vi "Actor Core.vi"(8 "error in":errorcluster, 11 "Nested in":refnum<class "Model_AMC.lvclass">) -> (0 "error out":errorcluster, 3 "Actor out":refnum<class "Actor.lvclass">)   [LabVIEW 2021, in "Model_AMC.lvclass"]
doc: "(<B>Filename</B>: Actor Framework.lvlib:Actor.lvclass:Actor Core.vi)\n\nReceives messages to the actor, reacts to them, and initiates any error handling that may shut the actor down.\n\nDescendant classes may override this VI to append parallel tasks for the actor to complete while it handles messages. Overrides use the Call Parent Method node."
uses:
  Model_AMC.lvclass
  Model_AMC.lvclass/Model_AMC.ctl
  <vilib>/ActorFramework/Actor/Actor.lvclass
  <vilib>/ActorFramework/Stop Msg/Stop Msg.lvclass
  <userlib>/John_Lib/AMC_FW/AMC_FW.lvlib
  <userlib>/John_Lib/Control/Panel State.ctl
  <userlib>/John_Lib/OPCUA/OPCUA.lvclass
  57b1ff99-141e-4da6-9bdf-70ec06928c0d.vi
  14795f1b-d0b1-44de-8d07-189a26e8dea2.vi
  C:/Program Files (x86)/National Instruments/LabVIEW 2021/user.lib/John_Lib/AbstractActorTemplate/AbstractActorTemplate/UIActorTop.lvclass
  C:/Program Files (x86)/National Instruments/LabVIEW 2021/vi.lib/ActorFramework/Actor/Actor.lvclass
  C:/Program Files (x86)/National Instruments/LabVIEW 2021/project/Create Actor from Template/_Model_AMC/Model_AMC.lvclass
  6f5781f2-676e-4ccc-9b4e-d2ad4bb5011c.vi
  <userlib>/John_Lib/AbstractActorTemplate/AbstractActorTemplate/UIActorTop.lvclass
  dd6ce886-d6bc-4aa3-89ad-92228f1f1005.vi
  eab6dcde-6998-4829-8205-257228226865.vi
  bac1cae5-b367-464c-b2b6-145fd5ecb0f6.vi
  TopRef.ctl
  b524a0ae-aab8-42c6-9847-114de1d87e8e.vi
panel:
  in  "Close":bool
  in  "Initialize":bool
  out "Close OK status":bool
  out "Initialize OK status":bool
  out "Messages":string
  out "Read Error":bool
  out "ReadIndex":u32
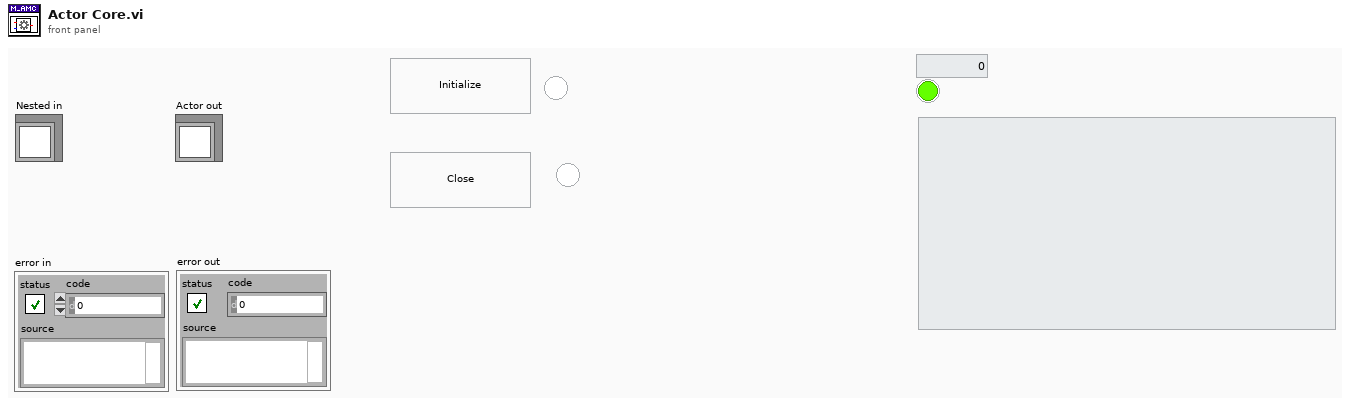
[diagram p1: front panel]
types:
  T1 = typedef "Model_AMC.lvclass/TopRef.ctl" = cluster{"Self ActorVI Ref":refnum<vi>}
  T2 = typedef "OPCUA.lvlib/OPCUA.lvclass/OPCUA Even.ctl" = cluster{"OPC UA data change":refnum<user-event>, "ReSubscribtion":refnum<user-event>}
  T3 = cluster{"Stop":refnum<user-event>, "Messages":refnum<user-event>}
  T4 = typedef "AMC_FW.lvlib/Queue.ctl" = cluster{"Q":T5, "Name":string}
  T5 = typedef "AMC_FW.lvlib/Message Queue.ctl" = refnum<queue>
  T6 = typedef "Panel State.ctl" = string
  T7 = typedef "Model_AMC.lvclass/DVR.ctl" = cluster{"JKI_Network_Streams":refnum<class "NetworkConnection.lvclass">, "AMC Q":T8, "Connnected":bool}
  T8 = typedef "Model_AMC.lvclass/AMC Q.ctl" = cluster{"Main":T4, "OPCUA":T4, "NetworkSteam":T4}
  T9 = typedef "AMC_FW.lvlib/Reply Data Type.ctl" = cluster{"Message Type":T10, "Data":variant}
  T10 = typedef "AMC_FW.lvlib/Message Type.ctl" = enum16{"Normal", "AMC_Reply", "OPCUA", "NetworkSteam"}
  T11 = typedef "Subscription Data Change.ctl" = cluster{"node ID":T12, " value":variant, "timestamp":timestamp, "data type":T13, "status code":T14}
  T12 = typedef "NodeId.ctl" = string
  T13 = typedef "Data Type.ctl" = u16
  T14 = typedef "OPC UA StatusCode.ctl" = u32
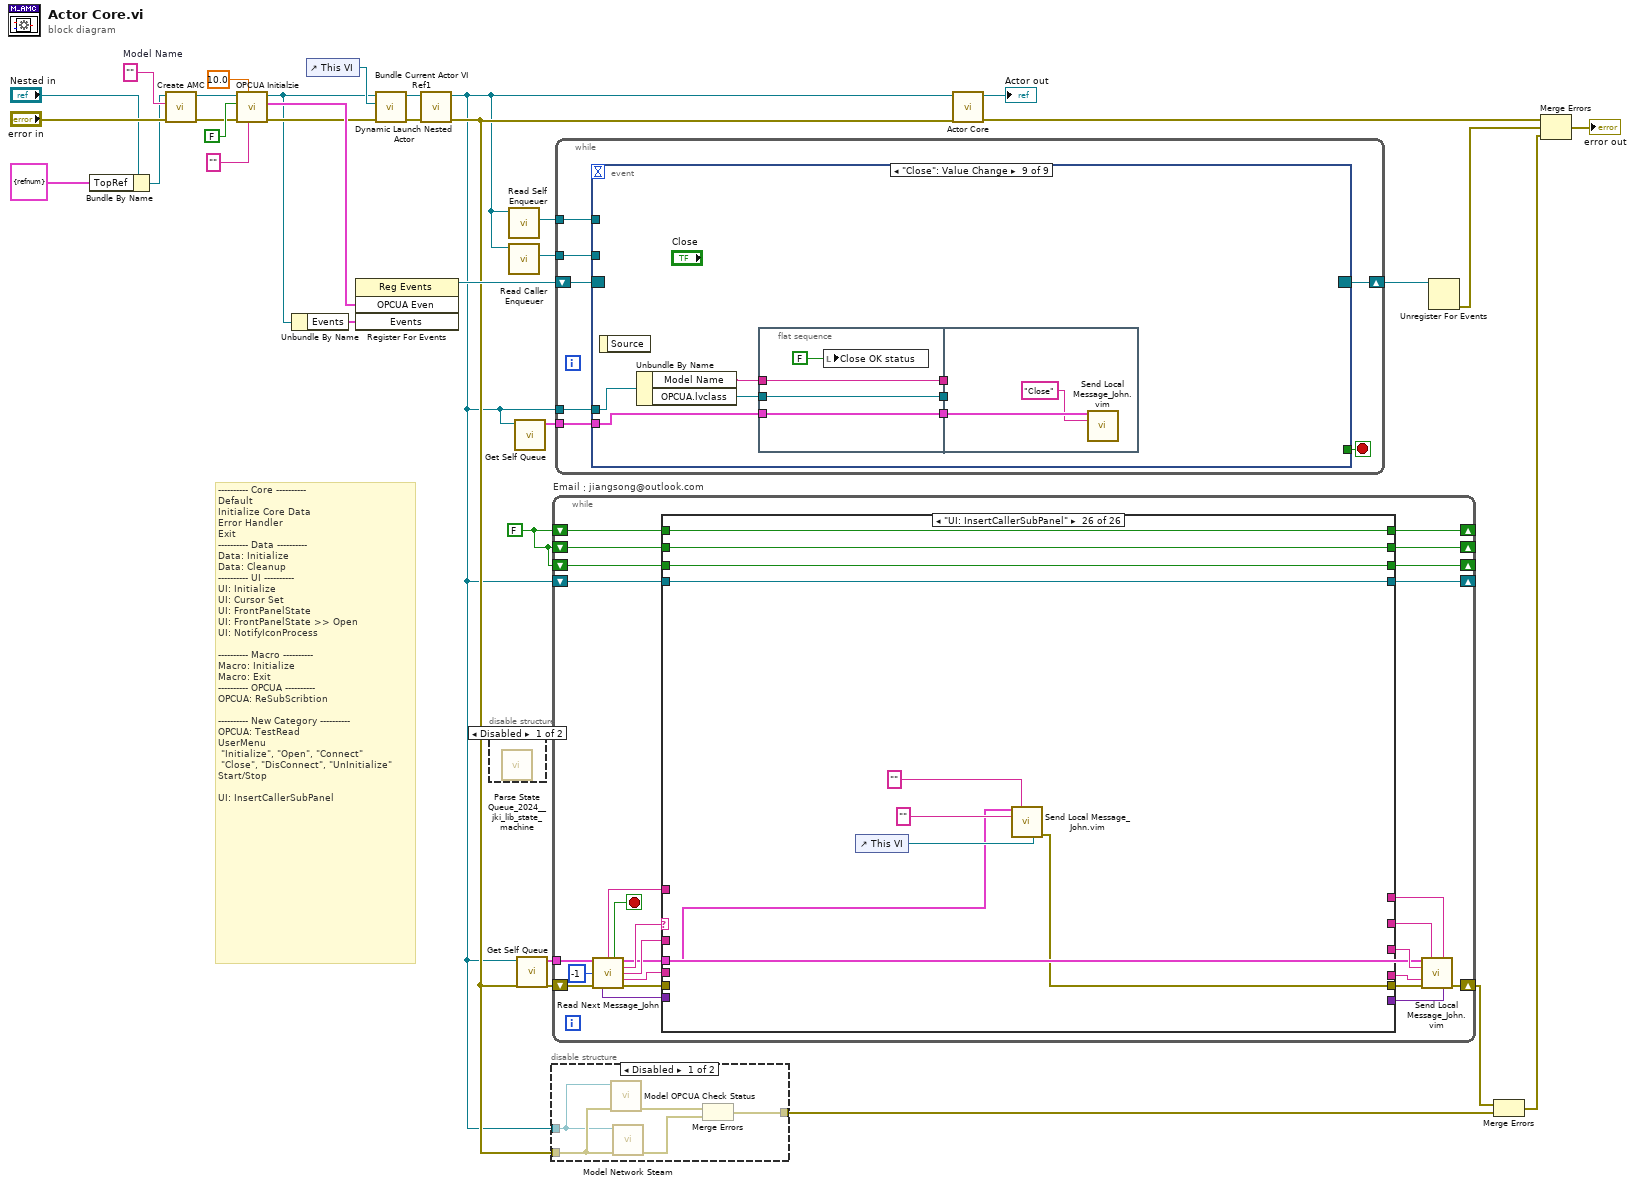
[diagram p0: block diagram]
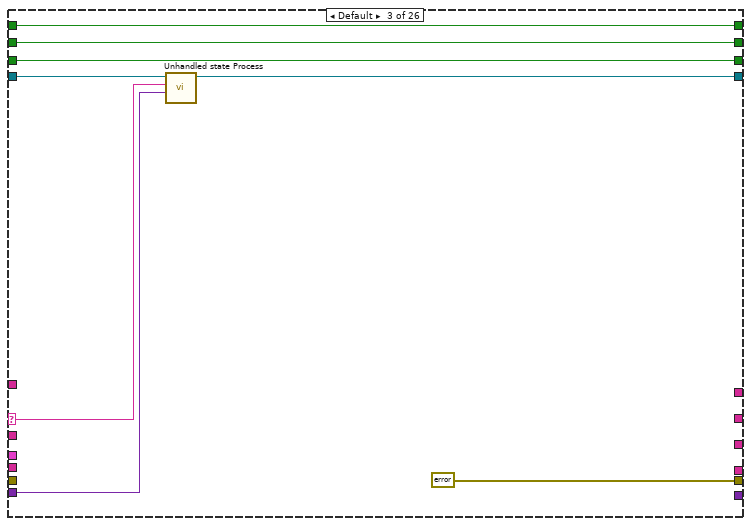
[diagram p6: hidden frame]
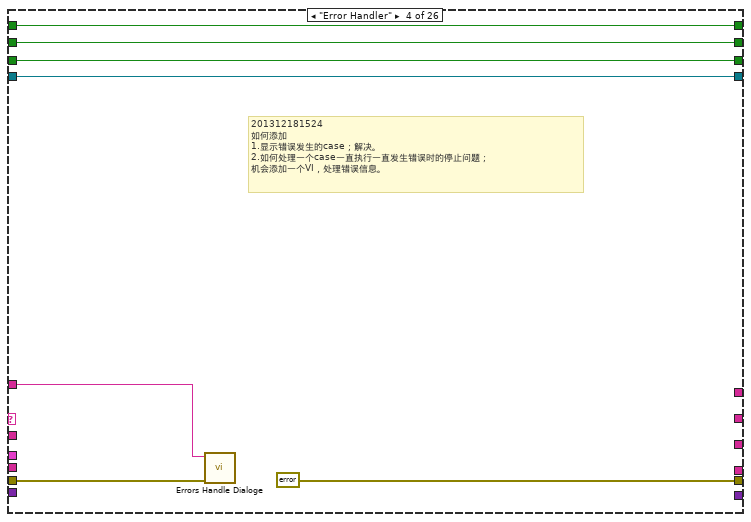
[diagram p7: hidden frame]
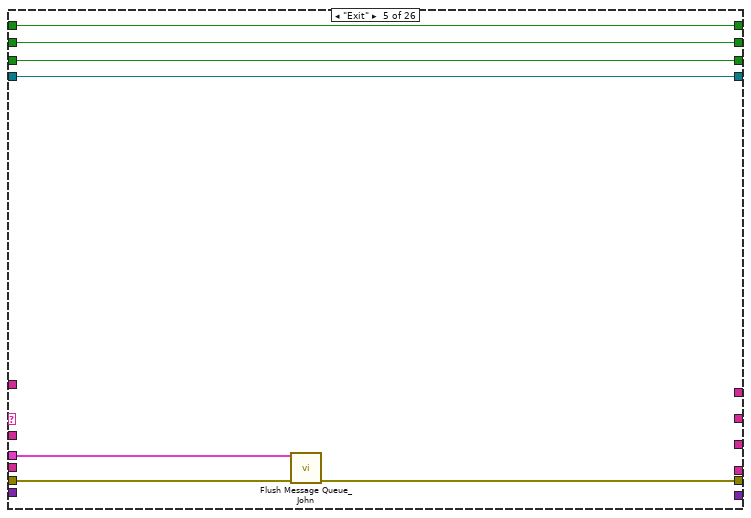
[diagram p8: hidden frame]
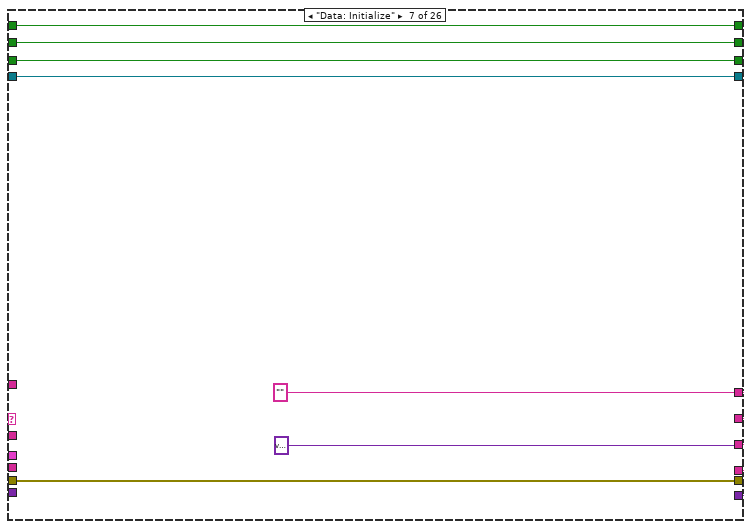
[diagram p10: hidden frame]
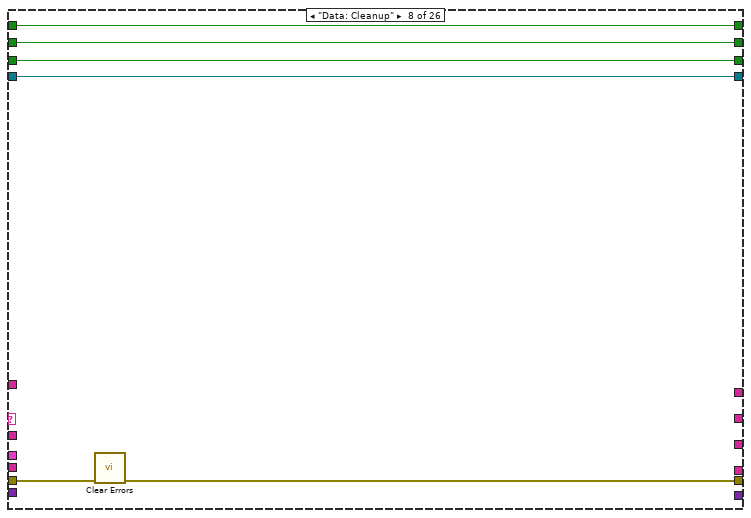
[diagram p11: hidden frame]
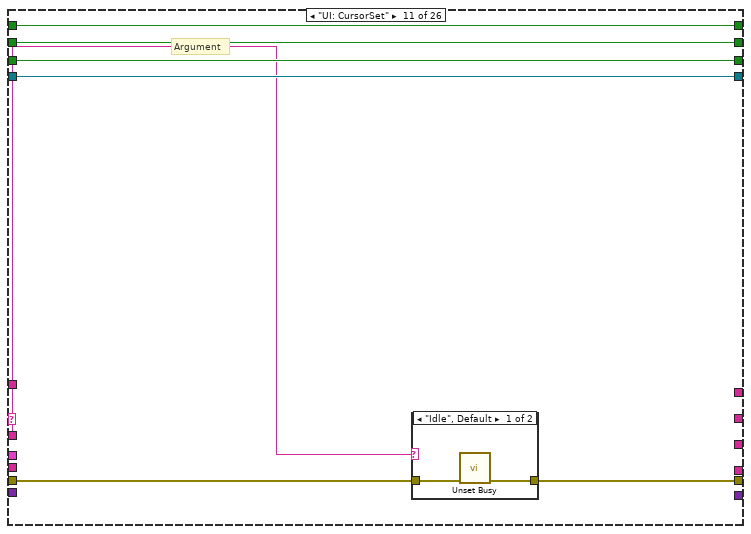
[diagram p14: hidden frame]
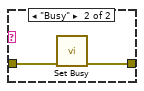
[diagram p15: hidden frame]
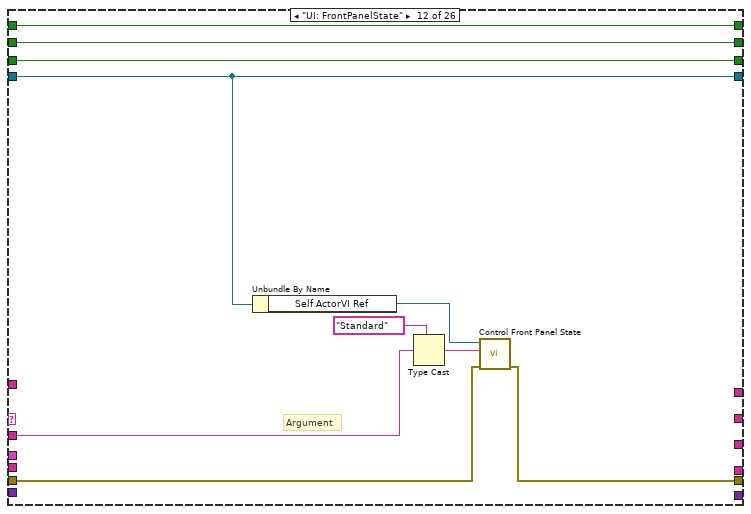
[diagram p16: hidden frame]
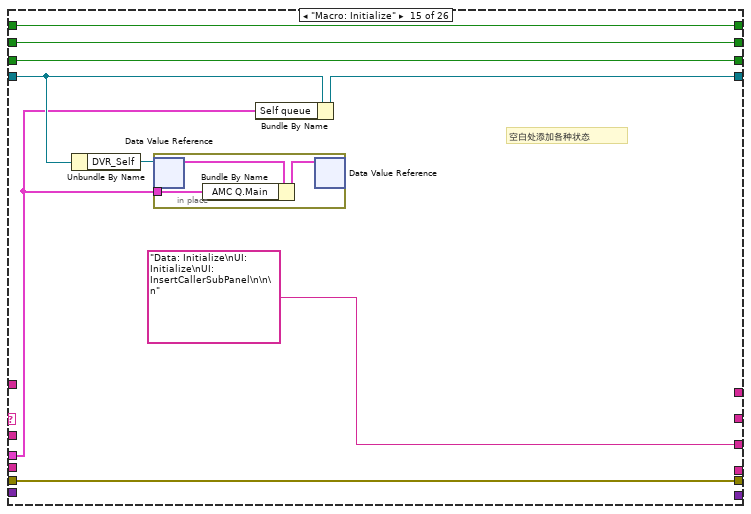
[diagram p19: hidden frame]
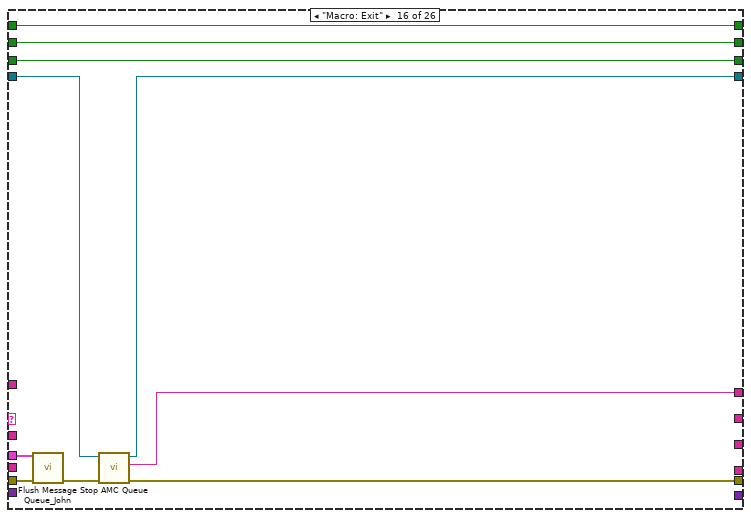
[diagram p20: hidden frame]
diagram:
  w18 = ""  # Model Name
  w25 = FALSE
  # "---------- Core ----------\nDefault\nInitialize Core Data\nError Handler\nExit\n---------- Data ----------\nData: Initialize\nData: Cleanup\n---------- UI ----------\nUI: Initialize\nUI: Cursor Set\nUI: FrontPanelState\nUI: FrontPanelState >> Open\nUI: NotifyIconProcess\n\n---------- Macro ----------\nMacro: Initialize\nMacro: Exit\n---------- OPCUA ----------\nOPCUA: ReSubScribtion\n\n---------- New Category ----------\nOPCUA: TestRead\nUserMenu\n \"Initialize\", \"Open\", \"Connect\" \n \"Close\", \"DisConnect\", \"UnInitialize\" \nStart/Stop\n\nUI: InsertCallerSubPanel"
  n1 = Bundle By Name(cluster="Nested in", "TopRef"=T1 {"Self ActorVI Ref"=refnum}) -> (w1:refnum<class "Model_AMC.lvclass">)
  n2 = call "Create AMC.vi"("error in (no error)"="error in", "message queue name"=w18, "Model_AMC in"=w1) -> ("error out"=w19:errorcluster, "Model_AMC out"=w21:refnum<class "Model_AMC.lvclass">)  [unwired: 7 in]
  n3 = call "OPCUA Initialzie.vi"("SUbscription Node IDs"="", "publishing interval (10 ms)"=10.0, "error in (no error)"=w19, "OPCUA Initialize"=FALSE, "Model_AMC in"=w21) -> ("error out"=w6:errorcluster, "OPCUA Even"=w17:T2, "Model_AMC out"=w3:refnum<class "Model_AMC.lvclass">)  [unwired: 4 in]
  n4 = Unbundle By Name(w3) -> ("Events"=w9:T3)
  n5 = control-ref of="This VI"() -> (w7:refnum<vi>)
  n6 = register-events ("Main Register for Events")(w17, w9) -> (reference out=w32:refnum<event-registration>)  [unwired: 2 in, 1 out]
  n7 = call "Bundle Current Actor VI Ref1.vi"("error in (no error)"=w6, "This VI"=w7, "Model_AMC in"=w3) -> ("error out"=w5:errorcluster, "Model_AMC out"=w8:refnum<class "Model_AMC.lvclass">)  [unwired: 5 in, 2 out]
  n8 = call-dynamic "Dynamic Launch Nested Actor.vi"("error in (no error)"=w5, "UI ActorTop in"=w8) -> ("error out"=w24:errorcluster, "UI ActorTop out"=w13:refnum<class "Model_AMC.lvclass">)  [unwired: 8 in]
  n9 = disable-structure shown="Disabled" {
    frame Disabled {
      n10 = call <vilib>:"Parse State Queue_2024__jki_lib_state_machine.vi"() -> ()  [unwired: 12 in, 4 out]
    }
    frame Enabled {
    }
  }
  n11 = call <vilib>:"Read Self Enqueuer.vi"("Actor"=w13) -> ("Self Enqueuer"=w27:refnum<class "Message Enqueuer.lvclass">)  [unwired: 10 in]
  n12 = call <vilib>:"Read Caller Enqueuer.vi"("Actor"=w13) -> ("Caller Enqueuer"=w26:refnum<class "Message Enqueuer.lvclass">)  [unwired: 10 in]
  n13 = call "Get Self Queue.vi"("Model_AMC in"=w13) -> ("Self queue"=w12:T4)  [unwired: 10 in]
  n14 = call "Get Self Queue.vi"("Model_AMC in"=w13) -> ("Self queue"=w22:T4)  [unwired: 10 in]
  n15 = disable-structure shown="Disabled" {
    disable-tunnel: w24 -> [w38 _]
    disable-tunnel: w13 -> [w37 _]
    disable-tunnel: [w34 _] -> w16
    frame Disabled {
      n16 = call "Model OPCUA Check Status.vi"("error in (no error)"=w38, "Model_AMC in"=w37) -> ("error out"=w36:errorcluster)  [unwired: 8 in, 1 out]
      n17 = call "Model Network Steam.vi"("error in (no error)"=w38, "Model_AMC in"=w37) -> ("error out"=w35:errorcluster)  [unwired: 8 in, 1 out]
      n18 = Merge Errors(w36, w35) -> (w34:errorcluster)
    }
    frame Enabled {
    }
  }
  n19 = while "Email：jiangsong@outlook.com" {
    shift-right: [w49] -> w15
    shift-left: w24 -> [w58]
    shift-right: [w63] -> _
    shift-left: w25 -> [w64]
    shift-right: [w59] -> _
    shift-left: w13 -> [w52]
    shift-right: [w60] -> _
    shift-left: w25 -> [w50]
    shift-right: [w61] -> _
    shift-left: w25 -> [w62]
    tunnel: w22 -> [w55]
    stop <- w41 stop-if-true
    n20 = call <userlib>:"Read Next Message_John.vi"("Queue In"=w55, "timeout (-1 ms)"=-1, "error in"=w58) -> ("Previous State + Arguments"=w51:string, "exit process?"=w41:bool, "Queue Out"=w40:T4, "Current State"=w56:string, "Arguments"=w54:string, "message value"=w53:string, "variant"=w42:variant, "error out"=w57:errorcluster)  [unwired: 3 in, 2 out]
    n21 = case shown="\"UI: InsertCallerSubPanel\"" w56 {
      selector: w56 -> [_ _ w76 _ _ _ _ _ _ _ _ _ _ _ _ _ _ _ _ _ w206 w223 w242 w256 _ _]
      tunnel: w40 -> [_ _ _ _ w91 _ _ _ _ _ _ _ _ _ w156 w174 _ _ _ _ _ _ _ _ _ w280]
      tunnel: w53 -> [_ _ _ _ _ _ _ _ _ _ _ _ _ _ _ _ _ _ w192 _ w205 w219 _ w255 w269 _]
      tunnel: [w65 w74 errorcluster {"status"=FALSE, "code"=0, "source"=""} ("error out") errorcluster {"status"=FALSE, "code"=0, "source"=""} ("error out") w92 w98 w106 w111 w116 w122 w127 w139 w146 w152 w161 w170 w180 w190 w196 w204 w211 w221 w247 w261 w270 w279] -> w48
      tunnel: w57 -> [w65 w74 _ w84 w93 w98 w106 w109 w116 w122 w128 w140 w146 w152 w161 w173 w180 w190 w196 w204 w207 w226 w243 w257 _ _]
      tunnel: w64 -> [w69 w73 w82 w89 w96 w101 w108 w112 w119 w124 w131 w145 w150 w155 w164 w177 w182 w189 w195 w203 w218 w241 w254 w268 w278 w287]
      tunnel: [w69 w73 w82 w89 w96 w101 w108 w112 w119 w124 w131 w145 w150 w155 w164 w177 w182 w189 w195 w203 w218 w241 w254 w268 w278 w287] -> w63
      tunnel: w62 -> [w68 w72 w81 w86 w95 w100 w107 w114 w118 w120 w130 w144 w149 w154 w163 w175 w181 w188 w194 w202 w217 w240 w253 w267 w277 w286]
      tunnel: w50 -> [w67 w70 w79 w87 w94 w97 w105 w110 w115 w121 w126 w143 w148 w151 w162 w176 w178 w187 w193 w201 w216 w239 w252 w266 w276 w285]
      tunnel: w52 -> [w66 w71 w77 w88 w90 w99 w103 w113 w117 w123 w129 w142 w147 w153 w157 w172 w179 w185 w191 w200 w212 w228 w248 w262 w273 w284]
      tunnel: [w68 w72 w81 w86 w95 w100 w107 w114 w118 w120 w130 w144 w149 w154 w163 w175 w181 w188 w194 w202 w217 w240 w253 w267 w277 w286] -> w61
      tunnel: [w67 w70 w79 w87 w94 w97 w105 w110 w115 w121 w126 w143 w148 w151 w162 w176 w178 w187 w193 w201 w216 w239 w252 w266 w276 w285] -> w60
      tunnel: [w66 w71 w78 w88 w90 w99 w103 w113 w117 w123 w129 w142 w147 w153 w159 w168 w179 w186 w191 w200 w213 w236 w249 w263 w271 w284] -> w59
      tunnel: w54 -> [_ _ _ _ _ _ _ _ _ _ w125 w136 _ _ _ _ _ _ _ _ _ _ _ _ _ _]
      tunnel: w51 -> [_ _ _ w83 _ _ _ _ _ _ _ _ _ _ _ _ _ _ _ _ _ _ _ _ _ _]
      tunnel: [_ _ _ _ _ _ w104 _ _ _ _ _ _ _ _ _ _ _ _ _ _ _ _ _ _ _] -> w47
      tunnel: [_ _ _ _ _ _ w104 _ _ _ _ _ _ _ _ w169 _ _ _ _ _ _ _ _ _ _] -> w46
      tunnel: [_ _ _ _ _ _ w104 _ _ _ _ _ _ _ "Data: Initialize\nUI: Initialize\nUI: InsertCallerSubPanel\n\n\n" _ _ _ _ _ _ w222 _ _ _ _] -> w45
      tunnel: [_ _ _ _ _ _ w104 _ _ _ _ _ _ _ _ _ _ _ _ _ _ _ _ _ _ _] -> w44
      tunnel: [_ _ _ _ _ _ variant ("variant") _ _ _ _ _ _ _ _ _ _ _ _ _ _ _ _ _ _ _] -> w43
      tunnel: w42 -> [_ _ w75 _ _ _ _ _ _ _ _ _ _ _ _ _ _ _ _ _ w215 w238 w251 w265 _ _]
      frame "", "Idle" {
      }
      frame "---------- Core ----------" {
      }
      frame Default {
        n22 = call "Unhandled state Process.vi"("variant"=w75, "Unhandled state Case Name"=w76, "Model_AMC in"=w77) -> ("Model_AMC out"=w78:refnum<class "Model_AMC.lvclass">)  [unwired: 7 in, 1 out]
      }
      frame "Error Handler" {
        # "201312181524\n如何添加\n1.显示错误发生的case；解决。\n2.如何处理一个case一直执行一直发生错误时的停止问题；\n机会添加一个VI，处理错误信息。"
        n23 = call <userlib>:"Errors Handle Dialoge.vi"("error in (no error)"=w84, "Message"=w83) -> ()  [unwired: 8 in, 2 out]
      }
      frame "Exit" {
        n24 = call <userlib>:"Flush Message Queue_John.vi"("Queue In"=w91, "error in"=w93) -> ("error out"=w92:errorcluster)  [unwired: 11 in, 2 out]
      }
      frame "---------- Data ----------" {
      }
      frame "Data: Initialize" {
        w104 = "" ("Elements in Front")
      }
      frame "Data: Cleanup" {
        n25 = call <vilib>:"Clear Errors.vi"("error in (no error)"=w109) -> ("error out"=w111:errorcluster)  [unwired: 5 in, 1 out]
      }
      frame "---------- UI ----------" {
      }
      frame "UI: Initialize" {
      }
      frame "UI: CursorSet" {
        # "Argument"
        n26 = case shown="\"Idle\", Default" w125 {
          tunnel: w128 -> [w133 w135]
          tunnel: [w132 w134] -> w127
          frame "Idle", Default {
            n27 = call <vilib>:"Unset Busy.vi"("error in (no error)"=w133) -> ("error out"=w132:errorcluster)  [unwired: 10 in]
          }
          frame "Busy" {
            n28 = call <vilib>:"Set Busy.vi"("error in (no error)"=w135) -> ("error out"=w134:errorcluster)  [unwired: 9 in, 1 out]
          }
        }
      }
      frame "UI: FrontPanelState" {
        # "Argument"
        n29 = Unbundle By Name(w142) -> ("Self ActorVI Ref"=w141:refnum<vi>)
        n30 = Type Cast(type=T6 "Standard" ("Argument"), x=w136) -> (*(type *) &x=w137:T6)
        n31 = call <userlib>:"Control Front Panel State.vi"("error out"=w140, "Argument"=w137, "Core.Current VI Reference"=w141) -> ("error out"=w139:errorcluster)  [unwired: 7 in, 1 out]
      }
      frame "UI: NotifyIconProcess" {
      }
      frame "---------- Macro ----------" {
      }
      frame "Macro: Initialize" {
        # "空白处添加各种状态"
        n32 = Unbundle By Name(w157) -> ("DVR_Self"=w158:refnum<data-value>)
        n33 = in-place {
          in-place-border: w156 -> [w165]
          n34 = in-place-dvr #1(w158) -> (w167:T7)  [unwired: 1 out]
          n35 = Bundle By Name(cluster=w167, "AMC Q.Main"=w165) -> (w166:T7)
          n36 = in-place-dvr #1(w166) -> ()  [unwired: 2 out]
        }
        n37 = Bundle By Name(cluster=w157, "Self queue"=w156) -> (w159:refnum<class "Model_AMC.lvclass">)
      }
      frame "Macro: Exit" {
        n38 = call <userlib>:"Flush Message Queue_John.vi"("Queue In"=w174, "error in"=w173) -> ("error out"=w171:errorcluster)  [unwired: 11 in, 2 out]
        n39 = call "Stop AMC Queue.vi"("error in (no error)"=w171, "Model_AMC in"=w172) -> ("error out"=w170:errorcluster, "Exist CMD"=w169:string, "Model_AMC out"=w168:refnum<class "Model_AMC.lvclass">)  [unwired: 7 in]
      }
      frame "---------- Control ----------" {
      }
      frame "OPCUA: ReSubScribtion" {
        n40 = Unbundle By Name(w185) -> ("OPCUA.lvclass"=w183:refnum<class "OPCUA.lvclass">)
        n41 = call <userlib>:"ReCreate Subscription.vi"("OPCUA in"=w183) -> ("OPCUA out"=w184:refnum<class "OPCUA.lvclass">)  [unwired: 7 in, 3 out]
        n42 = Bundle By Name(cluster=w185, "OPCUA.lvclass"=w184) -> (w186:refnum<class "Model_AMC.lvclass">)
      }
      frame "UserMenu" {
        n43 = case shown="\"Show Block Diagram\"" w192 {
          tunnel: w191 -> [_ w197]
          frame "False", Default {
          }
          frame "Show Block Diagram" {
            n44 = Unbundle By Name(w197) -> ("Self ActorVI Ref"=w199:refnum<vi>)
            n45 = property class="VI"(reference=w199, "BDWin.Open"=TRUE ("Block Diagram Window:Open")) -> ()  [unwired: 1 in, 2 out]
          }
        }
      }
      frame "OPCUA: TestRead" {
      }
      frame "Feedback Example" {
        n46 = call <userlib>:"Get Reply Data.vi"("Data"=w215) -> ("Reply Data Type"=w214:T9)  [unwired: 7 in, 3 out]
        n47 = call <vilib>:"Parse State Queue_2024__jki_lib_state_machine.vi"("State Queue"=w205) -> ()  [unwired: 11 in, 4 out]
        n48 = call "Build Feedback Message.vi"("error in (no error)"=w207, "Message"=w206) -> ("error out"=w208:errorcluster, "Feedback"=w209:string, "OK status"=w210:bool)  [unwired: 7 in]
        n49 = call "AMC Feedback Message.vi"("Result"=w210, "error in (no error)"=w208, "Messages"=w209, "Reply Data Type"=w214, "Model_AMC in"=w212) -> ("error out"=w211:errorcluster, "Model_AMC out"=w213:refnum<class "Model_AMC.lvclass">)  [unwired: 5 in]
      }
      frame "Connect", "Create", "Initialize", "Open" {
        n50 = call <vilib>:"Parse State Queue_2024__jki_lib_state_machine.vi"("State Queue"=w219) -> ()  [unwired: 11 in, 4 out]
        n51 = call <userlib>:"Get Reply Data.vi"("Data"=w238) -> ("Reply Data Type"=w237:T9)  [unwired: 7 in, 3 out]
        n52 = call "Error Dealy.vim"("value in"=w226, "milliseconds to wait"=u32 2000) -> ("value out"=w224:errorcluster)  [unwired: 1 out]
        n53 = Bundle By Name(cluster=w228, "ReadIndex"=u32 0) -> (w229:refnum<class "Model_AMC.lvclass">)
        n54 = Select(t=w223, s=w224, f="") -> (s? t:f=w222:string)
        n55 = call "DVR Update Connected.vi"("Connected"=FALSE, "Model_AMC in"=w229) -> ("Model_AMC out"=w232:refnum<class "Model_AMC.lvclass">)  [unwired: 8 in, 1 out]
        n56 = call "Build Feedback Message.vi"("error in (no error)"=w226, "Message"=w223) -> ("error out"=w233:errorcluster, "Feedback"=w234:string, "OK status"=w235:bool)  [unwired: 7 in]
        n57 = call "AMC Feedback Message.vi"("Result"=w235, "error in (no error)"=w233, "Messages"=w234, "Reply Data Type"=w237, "Model_AMC in"=w232) -> ("error out"=w220:errorcluster, "Model_AMC out"=w236:refnum<class "Model_AMC.lvclass">)  [unwired: 5 in]
        n58 = call <vilib>:"Clear Errors.vi"("error in (no error)"=w220) -> ("error out"=w221:errorcluster)  [unwired: 5 in, 1 out]
      }
      frame "Close", "DisConnect", "UnInitialize" {
        n59 = call <userlib>:"Get Reply Data.vi"("Data"=w251) -> ("Reply Data Type"=w250:T9)  [unwired: 7 in, 3 out]
        n60 = call "Build Feedback Message.vi"("error in (no error)"=w243, "Message"=w242) -> ("error out"=w244:errorcluster, "Feedback"=w245:string, "OK status"=w246:bool)  [unwired: 7 in]
        n61 = call "AMC Feedback Message.vi"("Result"=w246, "error in (no error)"=w244, "Messages"=w245, "Reply Data Type"=w250, "Model_AMC in"=w248) -> ("error out"=w247:errorcluster, "Model_AMC out"=w249:refnum<class "Model_AMC.lvclass">)  [unwired: 5 in]
      }
      frame "Start", "Start-Stop", "Start/Stop", "Stop" {
        n62 = call <vilib>:"Parse State Queue_2024__jki_lib_state_machine.vi"("State Queue"=w255) -> ()  [unwired: 11 in, 4 out]
        n63 = call <userlib>:"Get Reply Data.vi"("Data"=w265) -> ("Reply Data Type"=w264:T9)  [unwired: 7 in, 3 out]
        n64 = call "Build Feedback Message.vi"("error in (no error)"=w257, "Message"=w256) -> ("error out"=w258:errorcluster, "Feedback"=w259:string, "OK status"=w260:bool)  [unwired: 7 in]
        n65 = call "AMC Feedback Message.vi"("Result"=w260, "error in (no error)"=w258, "Messages"=w259, "Reply Data Type"=w264, "Model_AMC in"=w262) -> ("error out"=w261:errorcluster, "Model_AMC out"=w263:refnum<class "Model_AMC.lvclass">)  [unwired: 5 in]
      }
      frame "Read" {
        n66 = call <vilib>:"Parse State Queue_2024__jki_lib_state_machine.vi"("State Queue"=w269) -> ()  [unwired: 11 in, 4 out]
        n67 = call "Read Data.vi"("Model_AMC in"=w273) -> ("error out"=w270:errorcluster, "Model_AMC out"=w272:refnum<class "Model_AMC.lvclass">)  [unwired: 9 in]
        n68 = Unbundle By Name(w272) -> ("ReadIndex"=→"ReadIndex":u32)
        n69 = Unbundle By Name(w270) -> ("status"=→"Read Error":bool)
        n70 = call "AMC Feedback Message.vi"("error in (no error)"=w270, "Model_AMC in"=w272) -> ("Model_AMC out"=w271:refnum<class "Model_AMC.lvclass">)  [unwired: 8 in, 1 out]
      }
      frame "UI: InsertCallerSubPanel" {
        n71 = control-ref of="This VI"() -> (w282:refnum<vi>)
        n72 = call "Send Local Message_John.vim"("Queue In"=w280, "receiver process (\"\" - local)"="" ("Elements in Front"), "Elements at Back"="" ("Elements in Front"), "variant"=w282) -> ("error out"=w279:errorcluster)  [unwired: 9 in, 2 out]
      }
    }
    n73 = call "Send Local Message_John.vim"("Queue In"=w40, "receiver process (\"\" - local)"=w47, "Elements in Front"=w46, "Elements at Back"=w45, "message value"=w44, "error in"=w48, "variant"=w43) -> ("error out"=w49:errorcluster)  [unwired: 6 in, 2 out]
  }
  n74 = while {
    tunnel: w27 -> [w291]
    tunnel: w26 -> [w290]
    tunnel: w13 -> [w289]
    shift-right: [w292] -> w31
    shift-left: w32 -> [w294]
    tunnel: w12 -> [w288]
    stop <- w293 stop-if-true
    n75 = event "UI Events" shown="[8] \"Close\": Value Change" {
      selector: w294 -> [_ _ _ _ _ _ _ _ _]
      dyn-events: [_ _ w306 _ _ _ _ _ _] -> w292
      timeout: _ -> [_ _ _ _ _ _ _ _ _]
      tunnel: [TRUE _ _ _ _ _ _ _ _] -> w293
      tunnel: w291 -> [_ _ _ _ _ w315 _ _ _]
      tunnel: w290 -> [_ _ _ _ _ _ _ _ _]
      tunnel: w289 -> [w298 w300 w307 _ w313 _ _ w322 w336]
      tunnel: w288 -> [_ _ _ _ _ _ _ w318 w333]
      event User Event {
        n76 = event-data() -> ()  [unwired: 1 in, 1 out]
        n77 = Unbundle By Name(w298) -> ("Self queue"=w297:T4)
        n78 = call "Send Local Message_John.vim"("Queue In"=w297, "Elements in Front"="Macro: Exit") -> ("error out"=w296:errorcluster)  [unwired: 11 in, 2 out]
        n79 = call <vilib>:"Clear Errors.vi"("error in (no error)"=w296) -> ()  [unwired: 5 in, 2 out]
      }
      event User Event {
        n80 = event-data() -> ("data change"=w301:T11[])  [unwired: 1 in, 5 out]
        n81 = for {
          tunnel: w301 -> [w303] mode=indexing
          tunnel: w300 -> [w302]
          n82 = call "Data Change Process.vi"("data change"=w303, "Model_AMC in"=w302) -> ()  [unwired: 8 in, 2 out]
        }
      }
      event User Event {
        n83 = event-data() -> ()  [unwired: 1 in, 5 out]
        n84 = Unbundle By Name(w307) -> ("OPCUA.lvclass"=w308:refnum<class "OPCUA.lvclass">, "Events"=w304:T3)
        n85 = call <userlib>:"Read OPC Even.vi"("OPCUA in"=w308) -> ("OPCUA Even"=w305:T2)  [unwired: 8 in, 2 out]
        n86 = register-events(w305, w304) -> (reference out=w306:refnum<event-registration>)  [unwired: 2 in, 1 out]
      }
      event Menu Activation? {
        n87 = event-data() -> ("MenuRef"=w309:refnum<k9>)  [unwired: 1 in, 4 out]
        n88 = disable-structure shown="Disabled" {
          disable-tunnel: w309 -> [w310 _]
          frame Disabled {
            n89 = call "Create Menu.vi"("Menu in"=w310) -> ()  [unwired: 10 in, 1 out]
          }
          frame Enabled {
          }
        }
        n90 = event-data() -> ()  [unwired: 2 in, 1 out]
      }
      event Menu Selection (User) {
        n91 = event-data() -> ("ItemTag"=w311:string)  [unwired: 1 in, 2 out]
        n92 = Unbundle By Name(w313) -> ("Self queue"=w312:T4)
        n93 = call "Send Local Message_John.vim"("Queue In"=w312, "Elements at Back"="UserMenu", "message value"=w311) -> ()  [unwired: 10 in, 3 out]
      }
      event Panel Close? {
        n94 = event-data() -> ()  [unwired: 1 in, 1 out]
        n95 = call <vilib>:"Send Normal Stop.vi"("Message Enqueuer"=w315) -> ()  [unwired: 10 in, 1 out]
        n96 = event-data("Discard?"=TRUE) -> ()  [unwired: 1 in, 1 out]
      }
      event "Messages": Value Change {
        n97 = event-data() -> ("NewVal"=→"Messages":string)  [unwired: 1 in, 5 out]
      }
      event "Initialize": Value Change {
        n98 = event-data() -> ()  [unwired: 1 in, 1 out]
        n99 = Unbundle By Name(w322) -> ("Model Name"=w320:string, "OPCUA.lvclass"=w323:refnum<class "OPCUA.lvclass">)
        n100 = flat-sequence {
          tunnel: w323 -> [w329]
          tunnel: [w329] -> w324
          tunnel: [w326] -> w321
          tunnel: w320 -> [w326]
          tunnel: [w325] -> w319
          tunnel: w318 -> [w325]
          tunnel: w324 -> [_]
          tunnel: w321 -> [_]
          tunnel: w319 -> [w331]
          frame #0 {
            n101 = local write "Initialize OK status"(FALSE ("Initialize OK status")) -> ()
            n102 = local write "Messages"("" ("Message")) -> ()
          }
          frame #1 {
            n103 = call "Send Local Message_John.vim"("Queue In"=w331, "Elements at Back"="Initialize") -> ()  [unwired: 11 in, 3 out]
          }
        }
      }
      event "Close": Value Change {
        n104 = event-data() -> ()  [unwired: 1 in, 1 out]
        n105 = Unbundle By Name(w336) -> ("Model Name"=w334:string, "OPCUA.lvclass"=w337:refnum<class "OPCUA.lvclass">)
        n106 = flat-sequence {
          tunnel: w337 -> [w342]
          tunnel: [w342] -> w338
          tunnel: [w340] -> w335
          tunnel: w334 -> [w340]
          tunnel: w333 -> [w339]
          tunnel: [w339] -> w332
          tunnel: w338 -> [_]
          tunnel: w335 -> [_]
          tunnel: w332 -> [w344]
          frame #0 {
            n107 = local write "Close OK status"(FALSE ("Initialize OK status")) -> ()
          }
          frame #1 {
            n108 = call "Send Local Message_John.vim"("Queue In"=w344, "Elements at Back"="Close") -> ()  [unwired: 11 in, 3 out]
          }
        }
      }
    }
  }
  n109 = call-parent "Actor Core.vi"("error in"=w24, "Actor in"=w13) -> ("error out"=w29:errorcluster, "Actor out"=→"Actor out":refnum<class "Actor.lvclass">)  [unwired: 8 in]
  n110 = Unregister For Events(event registration refnum=w31) -> (error out=w30:errorcluster)  [unwired: 1 in]
  n111 = Merge Errors(w15, w16) -> (w14:errorcluster)
  n112 = Merge Errors(w29, w30, w14) -> (→"error out":errorcluster)
